vi "LRelu.vi"(2 "Z":dbl) -> (0 "LRelu(Z)":dbl)   [LabVIEW 2020]
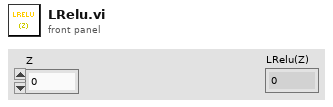
[diagram p1: front panel]
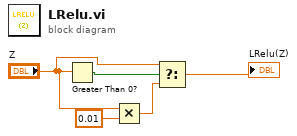
[diagram p0: block diagram]
diagram:
  n1 = Greater Than 0?(x="Z") -> (x > 0?=w4:bool)
  n2 = Multiply(x="Z", y=0.01) -> (x*y=w3:dbl)
  n3 = Select(t="Z", s=w4, f=w3) -> (s? t:f=→"LRelu(Z)":dbl)
